vi "Main On Compile Action VI_Parse Configuration.vi"(8 "error in (no error)":errorcluster, 11 "Item Ref in":T1 format="%.0x") -> (0 "error out":errorcluster, 2 "Channels":T2[](array[typedef]) {"RTs"."Mode Codes"."Words Item Refs" format="%.0x"; "RTs"."Mode Codes"."Timestamp Channel Data Reference" format="%.0x"; "RTs"."subAddresses"."Words Item Refs" format="%.0x"; "RTs"."subAddresses"."Timestamp Channel Data Reference" format="%.0x"; "RTs"."Status Channel Data Reference" format="%.0x"; "RTs"."Command Channels Refs" format="%.0x"; "BC"."Acyclic Frames Trigger Channels Refs" format="%.0x"; "BC"."Command Channels Refs" format="%.0x"; "BC"."messages"."Timestamp Channel Data Reference" format="%.0x"; "BC"."messages"."Status Channel Data Refs" format="%.0x"; "BC"."messages"."Words Item Refs" format="%.0x"; "BC"."messages"."Words Block Data Refs"."Data Reference" format="%.0x"}, 3 "Section Ref out":T1 format="%.0x")   [LabVIEW 2017, in "Ballard 1553 System Explorer.lvlib"]
uses:
  Ballard 1553 System Explorer.lvlib
  Shared/Controls and Global/RT Channel.ctl
  Shared/Controls and Global/RT BC.ctl
  <vilib>/NI Veristand/Custom Device API/Custom Device Item Ref.ctl
  Shared/Controls and Global/RT Message.ctl
  Shared/Controls and Global/RT messageType.ctl
  Shared/Controls and Global/RT CWD1.ctl
  Shared/Controls and Global/RT CWD2.ctl
  <vilib>/NI Veristand/Custom Device API/Data Reference.ctl
  <vilib>/NI Veristand/Custom Device API/Block Data Reference.ctl
  Shared/Controls and Global/RT Remote Terminal.ctl
  Shared/Controls and Global/RT Remote Terminal_rtMode.ctl
  Shared/Controls and Global/RT Remote Terminal_RT subAddress.ctl
  Shared/Controls and Global/RT Remote Terminal_RT direction.ctl
  Shared/Controls and Global/RT Remote Terminal_RT Mode Code.ctl
  <vilib>/NI Veristand/Custom Device API/Get Item Property (U16).vi
  <vilib>/NI Veristand/Custom Device Tools/Custom Device Utility Library/NI VeriStand - Search for All Items by GUID.vi
  <vilib>/NI Veristand/Custom Device API/Get Item Property (Boolean).vi
  Shared/Controls and Global/Global.vi
  Shared/Ballard 1553 Shared.lvlib
  <vilib>/NI VeriStand/Custom Device API/Custom Device API.lvlib
  <vilib>/NI VeriStand/Custom Device Tools/Custom Device Utility Library/Custom Device Utility Library.lvlib
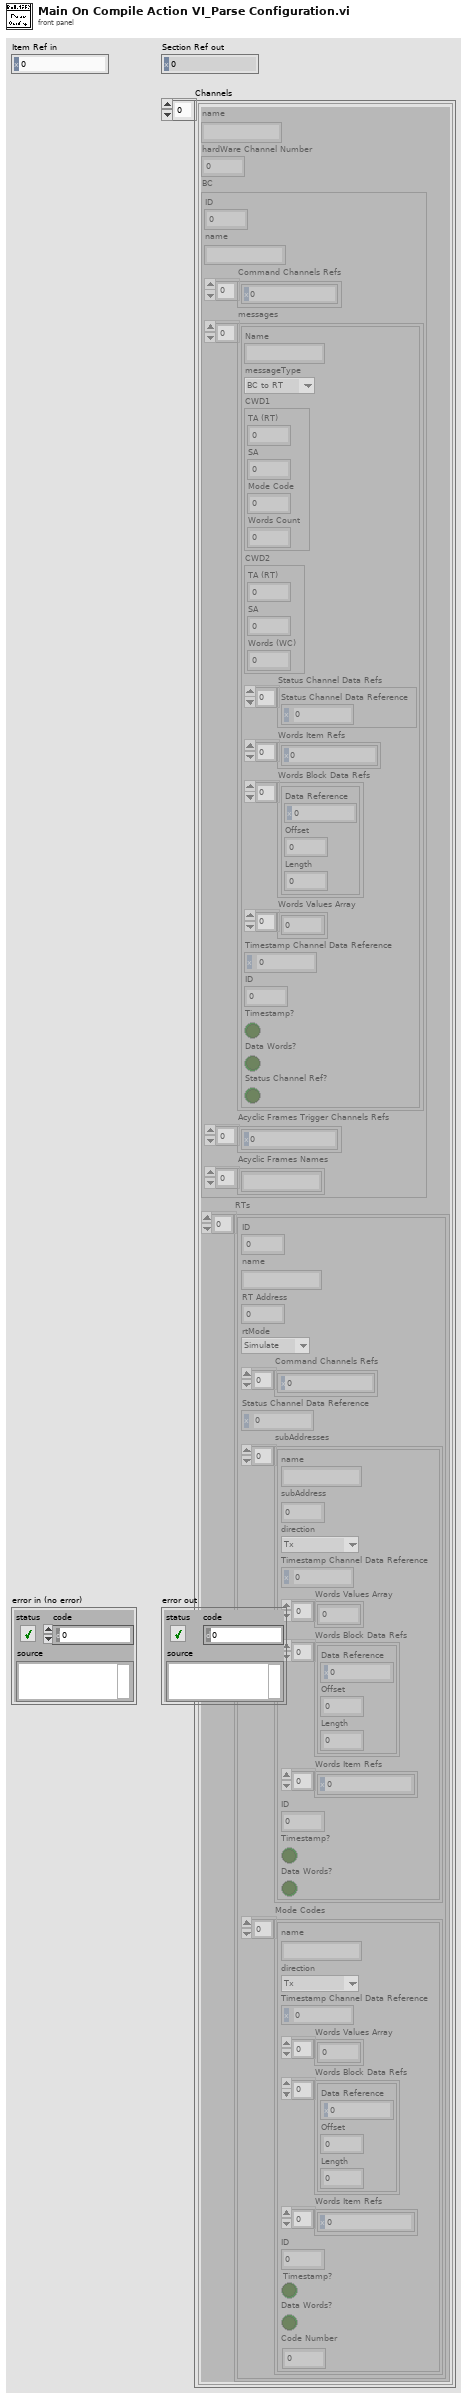
[diagram p1: front panel]
types:
  T1 = typedef "Custom Device API.lvlib/Custom Device Item Ref.ctl" = u64
  T2 = typedef "Ballard 1553 Shared.lvlib/RT Channel.ctl" = cluster{"name":string, "hardWare Channel Number":u16, "BC":T3, "RTs":T10[]}
  T3 = typedef "Ballard 1553 Shared.lvlib/RT BC.ctl" = cluster{"ID":i32, "name":string, "Command Channels Refs":T1[], "messages":T4[], "Acyclic Frames Trigger Channels Refs":T1[], "Acyclic Frames Names":string[]}
  T4 = typedef "Ballard 1553 Shared.lvlib/RT Message.ctl" = cluster{"Name":string, "messageType":T5, "CWD1":T6, "CWD2":T7, "Status Channel Data Refs":T8[], "Words Item Refs":T1[], "Words Block Data Refs":T9[], "Words Values Array":u16[], "Timestamp Channel Data Reference":T8, "ID":i32, "Timestamp?":bool, "Data Words?":bool, "Status Channel Ref?":bool}
  T5 = typedef "Ballard 1553 Shared.lvlib/RT messageType.ctl" = enum16{"BC to RT", "RT to BC", "RT to RT", "MC (Rx)", "MC (Tx)"}
  T6 = typedef "Ballard 1553 Shared.lvlib/RT CWD1.ctl" = cluster{"TA (RT)":i8, "SA":i8, "Mode Code":i8, "Words Count":i8}
  T7 = typedef "Ballard 1553 Shared.lvlib/RT CWD2.ctl" = cluster{"TA (RT)":i8, "SA":i8, "Words (WC)":i8}
  T8 = typedef "Custom Device API.lvlib/Data Reference.ctl" = i32
  T9 = typedef "Custom Device API.lvlib/Block Data Reference.ctl" = cluster{"Data Reference":T8, "Offset":u64, "Length":u64}
  T10 = typedef "Ballard 1553 Shared.lvlib/RT Remote Terminal.ctl" = cluster{"ID":i32, "name":string, "RT Address":i32, "rtMode":T11, "Command Channels Refs":T1[], "Status Channel Data Reference":T8, "subAddresses":T12[], "Mode Codes":T14[]}
  T11 = typedef "Ballard 1553 Shared.lvlib/RT Remote Terminal_rtMode.ctl" = enum16{"Simulate", "Monitor", "Disable"}
  T12 = typedef "Ballard 1553 Shared.lvlib/RT Remote Terminal_RT subAddress.ctl" = cluster{"name":string, "subAddress":i8, "direction":T13, "Timestamp Channel Data Reference":T8, "Words Values Array":u16[], "Words Block Data Refs":T9[], "Words Item Refs":T1[], "ID":i32, "Timestamp?":bool, "Data Words?":bool}
  T13 = typedef "Ballard 1553 Shared.lvlib/RT Remote Terminal_RT direction.ctl" = enum16{"Tx", "Rx"}
  T14 = typedef "Ballard 1553 Shared.lvlib/RT Remote Terminal_RT Mode Code.ctl" = cluster{"name":string, "direction":T13, "Timestamp Channel Data Reference":T8, "Words Values Array":u16[], "Words Block Data Refs":T9[], "Words Item Refs":T1[], "ID":i32, "Timestamp?":bool, "Data Words?":bool, "Code Number":i32}
  T15 = typedef "Custom Device API.lvlib/Custom Device Item Info.ctl" = cluster{"Name":string, "Is Channel":bool, "GUID":string, "Is Waveform":bool}
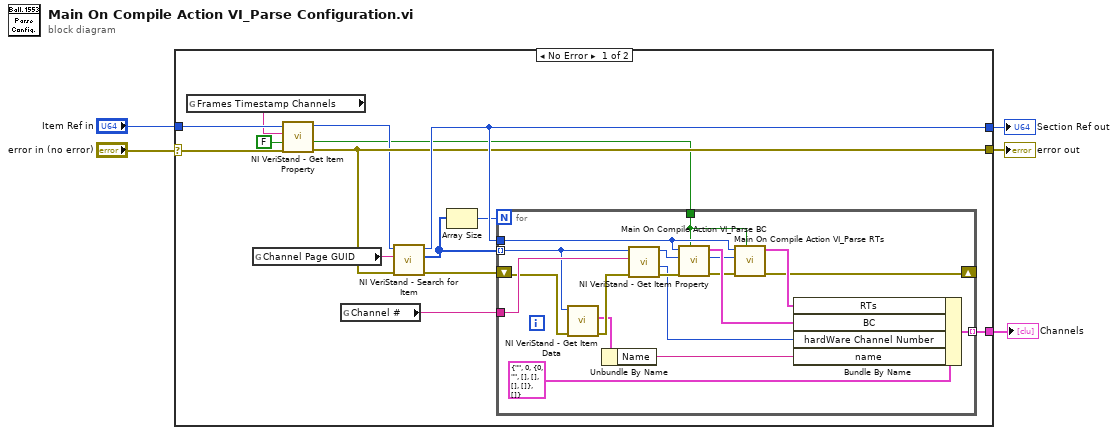
[diagram p0: block diagram]
diagram:
  n1 = case shown="No Error" "error in (no error)" {
    selector: "error in (no error)" -> [w6 w39]
    tunnel: [w19 _] -> w5
    tunnel: [w18 w38] -> w4
    tunnel: [w13 w39] -> w3
    tunnel: "Item Ref in" -> [w10 w38]
    frame No Error {
      n2 = global read "Global.vi" "Frames Timestamp Channels"() -> (w7:string)
      n3 = global read "Global.vi" "Channel Page GUID"() -> (w11:string)
      n4 = call-poly <vilib>:"NI VeriStand - Get Item Property.vi"("error in (no error)"=w6, "Default Value"=FALSE, "Property Name"=w7, "Item Ref in"=w10) -> ("error out"=w13:errorcluster, "Value"=w9:bool, "Item Ref out"=w12:T1)  [unwired: 4 in, 1 out]
      n5 = global read "Global.vi" "Channel #"() -> (w17:string)
      n6 = call-poly <vilib>:"NI VeriStand - Search for Item.vi"("error in"=w13, "Item GUID"=w11, "Section Ref in"=w12) -> ("error out"=w14:errorcluster, "Item Refs"=w16:T1[], "Section Ref out"=w18:T1)  [unwired: 5 in, 1 out]
      n7 = Array Size(array=w16) -> (size(s)=w15:i32)
      n8 = for {
        N: w15 -> [_]
        tunnel: w9 -> [w23]
        shift-right: [w20] -> _
        shift-left: w14 -> [w34]
        tunnel: w16 -> [w35] mode=indexing
        tunnel: w17 -> [w37]
        tunnel: w18 -> [w25]
        tunnel: [w26] -> w19 mode=indexing
        n9 = call <vilib>:"NI VeriStand - Get Item Data.vi"("error in (no error)"=w34, "Item Ref in"=w35) -> ("error out"=w33:errorcluster, "Item Info"=w32:T15)  [unwired: 6 in, 2 out]
        n10 = Unbundle By Name(w32) -> ("Name"=w31:string)
        n11 = call-poly <vilib>:"NI VeriStand - Get Item Property.vi"("error in (no error)"=w33, "Property Name"=w37, "Item Ref in"=w35) -> ("error out"=w36:errorcluster, "Value"=w29:u16, "Item Ref out"=w28:T1)  [unwired: 5 in, 1 out]
        n12 = call "Main On Compile Action VI_Parse BC.vi"("Autocreate Rx timestamp chans?"=w23, "error in"=w36, "Channel Ref"=w28, "Device Item Ref in"=w25) -> ("error out"=w21:errorcluster, "Channel Ref"=w24:u64, "BC"=w27:T3)  [unwired: 5 in]
        n13 = call "Main On Compile Action VI_Parse RTs.vi"("Autocreate Rx timestamp chans?"=w23, "error in"=w21, "Channel Ref"=w24, "Device Item Ref in"=w25) -> ("error out"=w20:errorcluster, "RTs"=w22:T10[])  [unwired: 6 in]
        n14 = Bundle By Name(cluster=T2 {"name"="", "hardWare Channel Number"=0, "BC"={"ID"=0, "name"="", "Command Channels Refs"=[], "messages"=[], "Acyclic Frames Trigger Channels Refs"=[], "Acyclic Frames Names"=[]}, "RTs"=[]} ("RT Channel"), "RTs"=w22, "BC"=w27, "hardWare Channel Number"=w29, "name"=w31) -> (w26:T2)
      }
    }
    frame Error {
    }
  }
  "Channels" <- w5
  "Section Ref out" <- w4
  "error out" <- w3
